vi "HGF_FGV_VisitByName.appendData2Variant.vi"(0 "initData":variant, 2 "nameArray":string[](array[string]), 5 "error in (no error)":errorcluster) -> (14 "dup initData":variant, 19 "error out":errorcluster)   [LabVIEW 2012, in "HGF_FGV.lvlib" / "HGF_FGV_VisitByName.lvclass"]
doc: "Append object initialization data to Variant as attribute."
uses:
  HGF_FGV_VisitByName.lvclass
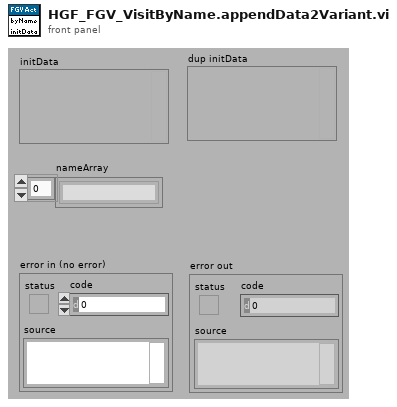
[diagram p1: front panel]
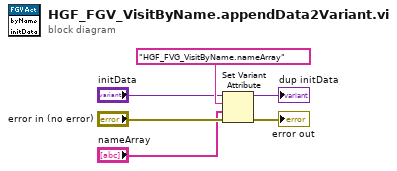
[diagram p0: block diagram]
diagram:
  n1 = Set Variant Attribute(Variant="initData", name="HGF_FVG_VisitByName.nameArray", value="nameArray", error in="error in (no error)") -> (Variant out=→"dup initData":variant, error out=→"error out":errorcluster)  [unwired: 1 out]
